vi "Data Count.vi"(8 "error in (no error)":errorcluster, 10 "Data Count":i32, 11 "Data Count Handler in":refnum<class "Data Count Handler.lvclass">) -> (0 "error out":errorcluster, 3 "Data Count Handler out":refnum<class "Data Count Handler.lvclass">)   [LabVIEW 2020, in "Scratchpad.lvlib" / "Test 1.lvlib" / "Data Count Handler.lvclass"]
uses:
  Data Count Handler.lvclass
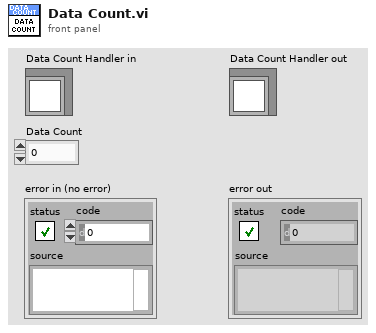
[diagram p1: front panel]
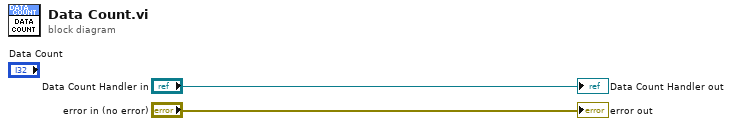
[diagram p0: block diagram]
diagram:
  "error out" <- "error in (no error)"
  "Data Count Handler out" <- "Data Count Handler in"
